vi "generate data for task.vi"(8 "error in (no error)":errorcluster, 11 "ImagingModeSPIM in":refnum<class "ImagingModeSPIM.lvclass">) -> (0 "error out":errorcluster, 2 "data to write":dbl, 3 "ImagingModeSPIM out":refnum<class "ImagingModeSPIM.lvclass">)   [LabVIEW 2012, in "ImagingModeSPIM.lvclass"]
uses:
  ImagingModeSPIM.lvclass
  ImagingModeSPIM.lvclass/ImagingModeSPIM.ctl
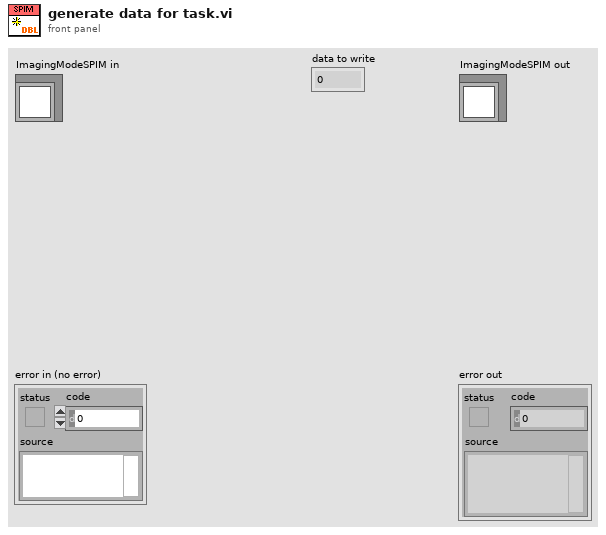
[diagram p1: front panel]
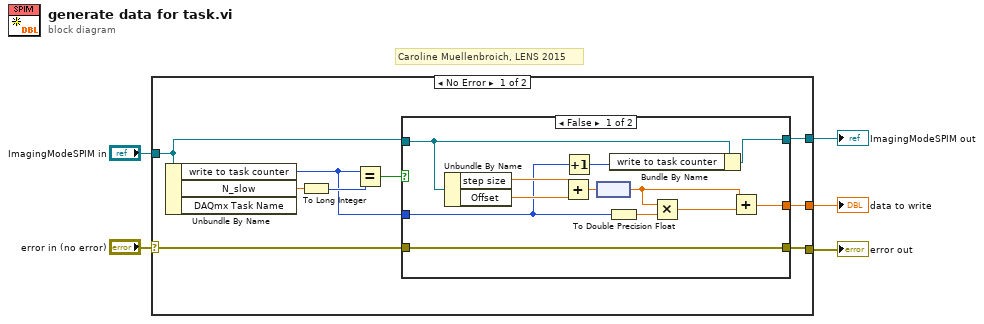
[diagram p0: block diagram]
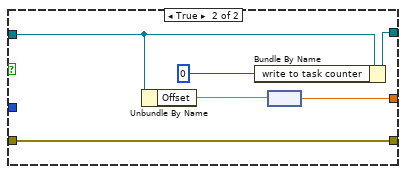
[diagram p2: hidden frame]
diagram:
  # "Caroline Muellenbroich, LENS 2015"
  n1 = case shown="No Error" "error in (no error)" {
    selector: "error in (no error)" -> [w8 w34]
    tunnel: [w7 w34] -> w4
    tunnel: [w10 w33] -> w2
    tunnel: "ImagingModeSPIM in" -> [w11 w33]
    tunnel: [w9 _] -> w1
    frame No Error {
      n2 = Unbundle By Name(w11) -> ("write to task counter"=w6:i32, "N_slow"=w13:dbl)  [unwired: 1 out]
      n3 = To Long Integer(number=w13) -> (32bit integer=w14:i32)
      n4 = Equal?(x=w6, y=w14) -> (x = y?=w12:bool)
      n5 = case shown="False" w12 {
        tunnel: w11 -> [w17 w30]
        tunnel: [w16 w29] -> w10
        tunnel: [w23 w31] -> w9
        tunnel: w8 -> [w22 w27]
        tunnel: [w22 w27] -> w7
        tunnel: w6 -> [w15 _]
        frame False {
          n6 = Unbundle By Name(w17) -> ("step size"=w26:dbl[unit], "Offset"=w25:dbl[unit])
          n7 = Add(x=w26, y=w25) -> (x+y=w24:dbl[unit])
          n8 = Increment(x=w15) -> (x+1=w18:i32)
          n9 = node(w24) -> (w21:dbl)
          n10 = To Double Precision Float(number=w15) -> (double precision float=w20:dbl)
          n11 = Bundle By Name(cluster=w17, "write to task counter"=w18) -> (w16:refnum<class "ImagingModeSPIM.lvclass">)
          n12 = Multiply(x=w21, y=w20) -> (x*y=w19:dbl)
          n13 = Add(x=w21, y=w19) -> (x+y=w23:dbl)
        }
        frame True {
          n14 = Unbundle By Name(w30) -> ("Offset"=w32:dbl[unit])
          n15 = Bundle By Name(cluster=w30, "write to task counter"=0 ("runtime cluster.Task cluster.write to task counter")) -> (w29:refnum<class "ImagingModeSPIM.lvclass">)
          n16 = node(w32) -> (w31:dbl)
        }
      }
    }
    frame Error {
    }
  }
  "error out" <- w4
  "ImagingModeSPIM out" <- w2
  "data to write" <- w1
